vi "Normalize Vector PtByPt.vi"(4 "initialize":bool, 5 "sample length":i32=100, 6 "input data point":dbl format="%0.2f") -> (0 "error":i32, 1 "mean":dbl format="%0.2f", 2 "standard deviation":dbl format="%0.2f", 3 "Normalized Vector":dbl[](array[numeric]))   [LabVIEW 2017, in "NI_PtbyPt.lvlib"]
doc: "Normalizes <B>input data point</B> using the statistical profile (<B>mean</B>,<B>standard deviation</B>) to obtain a <B>Normalized Vector</B> whose statistical profile is (0,1)."
uses:
  <vilib>/ptbypt/NI_PtbyPt.lvlib
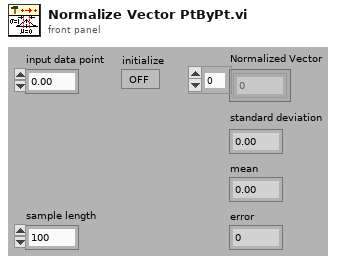
[diagram p1: front panel]
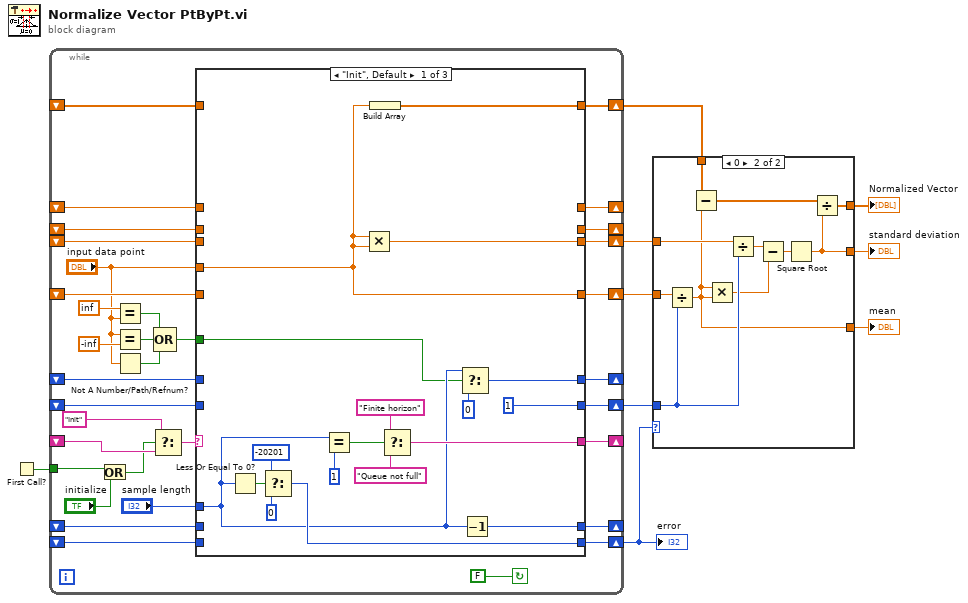
[diagram p0: block diagram]
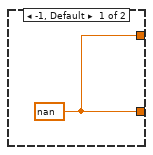
[diagram p2: hidden frame]
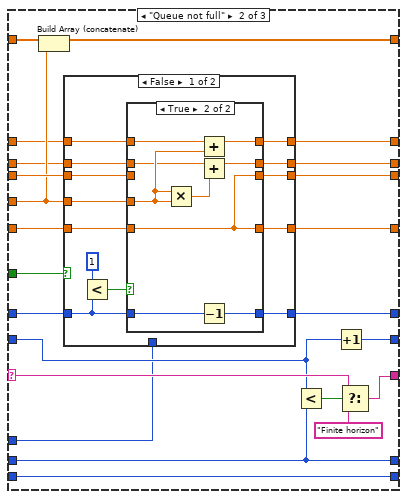
[diagram p3: hidden frame]
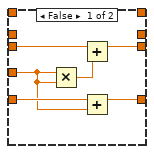
[diagram p4: hidden frame]
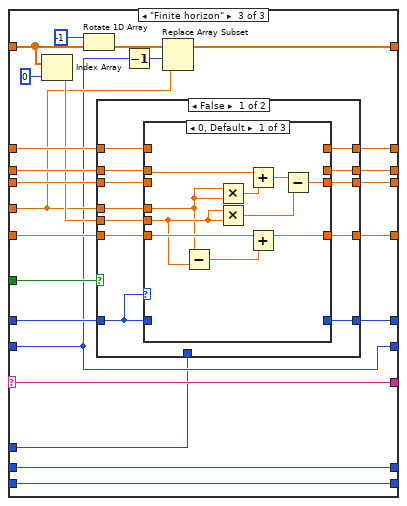
[diagram p6: hidden frame]
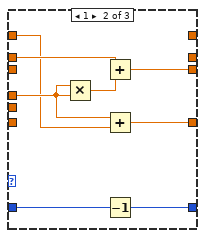
[diagram p7: hidden frame]
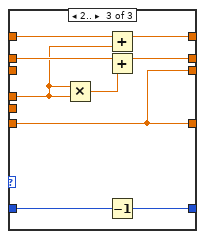
[diagram p8: hidden frame]
diagram:
  n1 = First Call?() -> (First Call?: T/F=w2:bool)
  n2 = while {
    tunnel: w2 -> [w27]
    shift-left: _ -> [w29]
    shift-right: [w30] -> w6
    shift-left: _ -> [w31]
    shift-right: [w32] -> _
    shift-left: _ -> [w34]
    shift-right: [w35] -> w9
    shift-left: _ -> [w37]
    shift-right: [w36] -> w4
    shift-left: _ -> [w39]
    shift-right: [w40] -> w5
    shift-left: _ -> [w43]
    shift-right: [w38] -> _
    shift-right: [w18] -> w1
    shift-left: _ -> [w17]
    shift-right: [w15] -> _
    shift-left: _ -> [w14]
    shift-right: [w13] -> _
    shift-left: _ -> [w12]
    shift-right: [w11] -> _
    shift-left: _ -> [w10]
    stop <- FALSE continue-if-true
    n3 = Or(x=w27, y="initialize") -> (x .or. y?=w25:bool)
    n4 = Equal?(x=inf, y="input data point") -> (x = y?=w21:bool)
    n5 = Equal?(x="input data point", y=-inf) -> (x = y?=w22:bool)
    n6 = Not A Number/Path/Refnum?(number/path/refnum="input data point") -> (NaN/Path/Refnum?=w20:bool)
    n7 = Select(t="Init", s=w25, f=w43) -> (s? t:f=w41:string)
    n8 = Compound Arithmetic op=OR(w21, w22, w20) -> (w16:bool)
    n9 = case shown="\"Init\", Default" w41 {
      selector: w41 -> [_ w65 w119]
      tunnel: "input data point" -> [w51 w78 w122]
      tunnel: [1 w77 w120] -> w40
      tunnel: w39 -> [_ w64 w120]
      tunnel: [w50 w66 w119] -> w38
      tunnel: w37 -> [_ w84 w125]
      tunnel: [w44 w83 w123] -> w36
      tunnel: "sample length" -> [w46 w62 w118]
      tunnel: [w53 w82 w137] -> w35
      tunnel: w34 -> [_ w81 w138]
      tunnel: [w52 w67 w136] -> w32
      tunnel: w31 -> [_ w67 w136]
      tunnel: [w51 w80 w134] -> w30
      tunnel: w29 -> [_ w79 w135]
      tunnel: [w49 w70 w129] -> w18
      tunnel: w17 -> [_ w70 w129]
      tunnel: w16 -> [w45 w63 w133]
      tunnel: [w47 w75 w117] -> w15
      tunnel: w14 -> [_ w76 w132]
      tunnel: [_ w74 w115] -> w13
      tunnel: w12 -> [_ w73 w130]
      tunnel: [_ w72 w116] -> w11
      tunnel: w10 -> [_ w71 w131]
      frame "Init", Default {
        n10 = Less Or Equal To 0?(x=w46) -> (x <= 0?=w54:bool)
        n11 = Select(t=-20201, s=w54, f=0) -> (s? t:f=w49:i32)
        n12 = Equal?(x=w46, y=1) -> (x = y?=w59:bool)
        n13 = Multiply(x=w51, y=w51) -> (x*y=w53:dbl)
        n14 = Build Array(w51) -> (w44:dbl[])
        n15 = Select(t="Finite horizon", s=w59, f="Queue not full") -> (s? t:f=w50:string)
        n16 = Select(t=w46, s=w45, f=0) -> (s? t:f=w47:i32)
        n17 = Decrement(x=w46) -> (x-1=w52:i32)
      }
      frame "Queue not full" {
        n18 = Build Array (concatenate)(w84, w78) -> (w83:dbl[])
        n19 = case shown="False" w63 {
          tunnel: [w97 w114] -> w82
          tunnel: w81 -> [w96 _]
          tunnel: [w95 w114] -> w80
          tunnel: w79 -> [w94 _]
          tunnel: w78 -> [w93 w114]
          tunnel: w76 -> [w92 _]
          tunnel: [w91 w113] -> w75
          tunnel: [w90 _] -> w74
          tunnel: w73 -> [w89 _]
          tunnel: [w88 _] -> w72
          tunnel: w71 -> [w87 _]
          tunnel: w62 -> [_ w113]
          frame False {
            n20 = Less?(x=1, y=w92) -> (x < y?=w85:bool)
            n21 = case shown="True" w85 {
              tunnel: [w103 w104] -> w97
              tunnel: w96 -> [w102 _]
              tunnel: [w100 w104] -> w95
              tunnel: w94 -> [w99 w104]
              tunnel: w93 -> [w98 w109]
              tunnel: w92 -> [_ w112]
              tunnel: [_ w111] -> w91
              tunnel: [_ w110] -> w90
              tunnel: w89 -> [_ w108]
              tunnel: [_ w106] -> w88
              tunnel: w87 -> [_ w105]
              frame False {
                n22 = Multiply(x=w98, y=w98) -> (x*y=w101:dbl)
                n23 = Add(x=w102, y=w101) -> (x+y=w103:dbl)
                n24 = Add(x=w99, y=w98) -> (x+y=w100:dbl)
              }
              frame True {
                n25 = Multiply(x=w109, y=w109) -> (x*y=w107:dbl)
                n26 = Add(x=w108, y=w109) -> (x+y=w110:dbl)
                n27 = Add(x=w105, y=w107) -> (x+y=w106:dbl)
                n28 = Decrement(x=w112) -> (x-1=w111:i32)
              }
            }
          }
          frame True {
          }
        }
        n29 = Less?(x=w64, y=w67) -> (x < y?=w68:bool)
        n30 = Increment(x=w64) -> (x+1=w77:i32)
        n31 = Select(t=w65, s=w68, f="Finite horizon") -> (s? t:f=w66:string)
      }
      frame "Finite horizon" {
        n32 = Index Array(array=w125, index=0 ("Index")) -> (element=w124:dbl)
        n33 = Rotate 1D Array(1:w125, 2:i16 -1 ("n")) -> (0:w127:dbl[])
        n34 = case shown="False" w133 {
          tunnel: w138 -> [w150 _]
          tunnel: [w149 w179] -> w137
          tunnel: w122 -> [w143 w179]
          tunnel: w135 -> [w148 _]
          tunnel: [w147 w179] -> w134
          tunnel: w132 -> [w139 _]
          tunnel: w131 -> [w146 _]
          tunnel: w130 -> [w145 _]
          tunnel: w124 -> [w144 _]
          tunnel: w118 -> [_ w178]
          tunnel: [w142 w178] -> w117
          tunnel: [w141 _] -> w116
          tunnel: [w140 _] -> w115
          frame False {
            n35 = case shown="0, Default" w139 {
              tunnel: w150 -> [w160 _ _]
              tunnel: [w156 w164 w169] -> w149
              tunnel: w143 -> [w151 w162 w175]
              tunnel: w148 -> [w155 _ w169]
              tunnel: [w154 w163 w169] -> w147
              tunnel: w146 -> [_ w168 w176]
              tunnel: w145 -> [_ w161 w177]
              tunnel: w144 -> [w152 _ _]
              tunnel: w139 -> [_ w167 w174]
              tunnel: [_ w166 w173] -> w142
              tunnel: [_ _ w170] -> w141
              tunnel: [_ _ w171] -> w140
              frame 0, Default {
                n36 = Subtract(x=w151, y=w152) -> (x-y=w153:dbl)
                n37 = Multiply(x=w151, y=w151) -> (x*y=w159:dbl)
                n38 = Multiply(x=w152, y=w152) -> (x*y=w157:dbl)
                n39 = Add(x=w160, y=w159) -> (x+y=w158:dbl)
                n40 = Add(x=w155, y=w153) -> (x+y=w154:dbl)
                n41 = Subtract(x=w158, y=w157) -> (x-y=w156:dbl)
              }
              frame 1 {
                n42 = Multiply(x=w162, y=w162) -> (x*y=w165:dbl)
                n43 = Add(x=w168, y=w165) -> (x+y=w164:dbl)
                n44 = Add(x=w162, y=w161) -> (x+y=w163:dbl)
                n45 = Decrement(x=w167) -> (x-1=w166:i32)
              }
              frame 2.. {
                n46 = Multiply(x=w175, y=w175) -> (x*y=w172:dbl)
                n47 = Add(x=w177, y=w175) -> (x+y=w171:dbl)
                n48 = Add(x=w176, y=w172) -> (x+y=w170:dbl)
                n49 = Decrement(x=w174) -> (x-1=w173:i32)
              }
            }
          }
          frame True {
          }
        }
        n50 = Decrement(x=w120) -> (x-1=w126:i32)
        n51 = Replace Array Subset(array=w127, new element=w122, index=w126) -> (w123:dbl[])
      }
    }
  }
  "error" <- w1
  n52 = case shown="0" w1 {
    tunnel: w9 -> [_ w190]
    tunnel: [_ w188] -> w8
    tunnel: [w180 w187] -> w7
    tunnel: w6 -> [_ w186]
    tunnel: w5 -> [_ w185]
    tunnel: w4 -> [_ w182]
    tunnel: [w180 w181] -> w3
    frame -1, Default {
      w180 = nan
    }
    frame 0 {
      n53 = Divide(x=w186, y=w185) -> (x/y=w181:dbl)
      n54 = Subtract(x=w182, y=w181) -> (x-y=w183:dbl[])
      n55 = Multiply(x=w181, y=w181) -> (x*y=w184:dbl)
      n56 = Divide(x=w190, y=w185) -> (x/y=w191:dbl)
      n57 = Subtract(x=w191, y=w184) -> (x-y=w189:dbl)
      n58 = Square Root(x=w189) -> (sqrt(x)=w187:dbl)
      n59 = Divide(x=w183, y=w187) -> (x/y=w188:dbl[])
    }
  }
  "mean" <- w3
  "Normalized Vector" <- w8
  "standard deviation" <- w7
